vi "VCF.vi"(7 "Amount":fxp<+,8,0>, 9 "Q1":fxp<+/-,18,18>, 10 "F1":fxp<+/-,18,18>, 11 "Sample In":fxp<+/-,8,8>) -> (1 "BP Out":fxp<+/-,8,8>, 2 "LP Out":fxp<+/-,8,8>, 3 "HP Out":fxp<+/-,8,8>)   [LabVIEW 2015]
doc: "Executes simultaneous LP, HP and BP point-by-point filtering, being able to modify both the cutoff frequency and the resonance at run time. It also enables growl control, by routing an envelope generator output to the 'Amount' input."
uses:
  <vilib>/rvi/FXPMathLib/basic elements/DSP48E/simVIs/niFpgaDsp48eSimulationState.ctl
  <vilib>/rvi/FXPMathLib/basic elements/DSP48E/subVIs/niFpgaDsp48eType.ctl
  <vilib>/rvi/FXPMathLib/basic elements/DSP48E/subVIs/niFpgaDsp48eAlumodeOpmodeCarryinselState.ctl
  <vilib>/rvi/FXPMathLib/basic elements/DSP48E/subVIs/niFpgaDsp48eUseMultiplierState.ctl
  <vilib>/rvi/FXPMathLib/basic elements/DSP48E/subVIs/niFpgaDsp48eLogicUnitModeState.ctl
  <vilib>/rvi/FXPMathLib/basic elements/DSP48E/subVIs/niFpgaDsp48eSelectPatternState.ctl
  <vilib>/rvi/FXPMathLib/basic elements/DSP48E/subVIs/niFpgaDsp48eSelectMaskState.ctl
  <vilib>/rvi/FXPMathLib/basic elements/DSP48E/subVIs/niFpgaDsp48eAutoresetState.ctl
  <vilib>/rvi/FXPMathLib/basic elements/DSP48E/simVIs/niFpgaDsp48eResets.ctl
  <vilib>/rvi/FXPMathLib/basic elements/DSP48E/simVIs/niFpgaDsp48eEnables.ctl
  <vilib>/rvi/FXPMathLib/basic elements/DSP48E/simVIs/niFpgaDsp48eRegisters.ctl
  <vilib>/rvi/FXPMathLib/basic elements/DSP48E/simVIs/niFpgaDsp48eCheckMode.vi
  <vilib>/rvi/FXPMathLib/basic elements/DSP48E/simVIs/niFpgaDsp48eReportInvalidMode.vi
  <vilib>/rvi/FXPMathLib/basic elements/DSP48E/simVIs/niFpgaDsp48eSimMultiplier.vi
  <vilib>/rvi/FXPMathLib/basic elements/DSP48E/simVIs/niFpgaDsp48eSimArithmetic.vi
  <vilib>/rvi/FXPMathLib/basic elements/DSP48E/simVIs/niFpgaDsp48eSimPatternDetect.vi
  <vilib>/rvi/FXPMathLib/basic elements/DSP48E/simVIs/niFpgaDsp48eSimP.vi
  <vilib>/rvi/FXPMathLib/basic elements/DSP48E/simVIs/niFpgaDsp48eSimUpdateState.vi
  <vilib>/rvi/FXPMathLib/FxpMul/XNode/nifxpmath_Multiplier.xnode
  <vilib>/rvi/FXPMathLib/basic elements/DSP48E/XNode/niFpgaDsp48e.xnode
  <vilib>/rvi/FXPMathLib/sim/FxpSim.dll
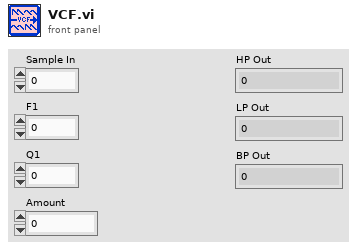
[diagram p1: front panel]
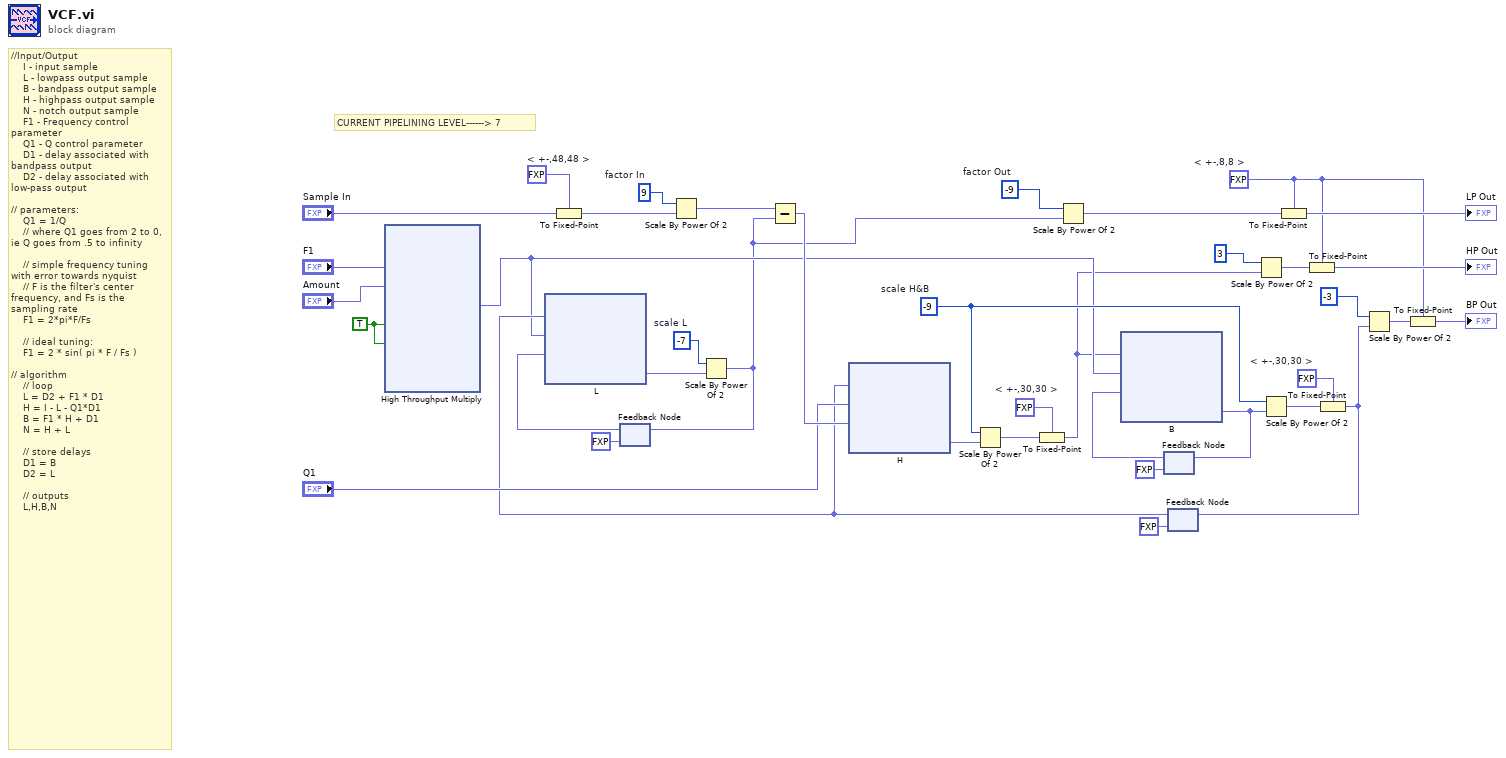
[diagram p0: block diagram]
diagram:
  w16 = TRUE ("input valid")
  w11 = i16 -9  # factor Out
  w19 = i16 -9  # scale H&B
  w32 = i16 -7  # scale L
  w30 = i16 9  # factor In
  w22 = fxp<+/-,30,30> 0.0  # < +-,30,30 >
  w24 = fxp<+/-,30,30> 0.0  # < +-,30,30 >
  w38 = fxp<+/-,48,48> 0.0  # < +-,48,48 >
  w1 = fxp<+/-,8,8> 0.0  # < +-,8,8 >
  # "CURRENT PIPELINING LEVEL------> 7"
  # "//Input/Output\n    I - input sample\n    L - lowpass output sample\n    B - bandpass output sample\n    H - highpass output sample\n    N - notch output sample\n    F1 - Frequency control parameter\n    Q1 - Q control parameter\n    D1 - delay associated with bandpass output\n    D2 - delay associated with low-pass output\n    \n// parameters:\n    Q1 = 1/Q \n    // where Q1 goes from 2 to 0, ie Q goes from .5 to infinity\n    \n    // simple frequency tuning with error towards nyquist\n    // F is the filter's center frequency, and Fs is the sampling rate\n    F1 = 2*pi*F/Fs\n\n    // ideal tuning:\n    F1 = 2 * sin( pi * F / Fs )\n\n// algorithm\n    // loop\n    L = D2 + F1 * D1\n    H = I - L - Q1*D1\n    B = F1 * H + D1\n    N = H + L\n    \n    // store delays\n    D1 = B\n    D2 = L\n\n    // outputs\n    L,H,B,N"
  n1 = xnode "High Throughput Multiply"("x"="F1", "y"="Amount", "input valid"=w16, "ready for output (T)"=w16) -> ("x*y"=w17:fxp<+/-,18,18>)  [unwired: 2 out]
  n2 = To Fixed-Point(fixed-point type=w38, number="Sample In") -> (fixed-point=w36:fxp<+/-,48,48>)
  n3 = feedback #1(fxp<+/-,48,48> 1.0) -> (w34:fxp<+/-,48,48>)
  n4 = Scale By Power Of 2(n=w30, x=w36) -> (x*2^n=w31:fxp<+/-,48,48>)
  n5 = feedback #2(fxp<+/-,48,48> 1.0 ("p")) -> (w27:fxp<+/-,48,48>)
  n6 = feedback #3(fxp<+/-,30,30> 1.0 ("< +-,30,30 >")) -> (w23:fxp<+/-,30,30>)
  n7 = xnode "L"("a"=w23, "b"=w17, "c"=w34) -> ("p"=w33:fxp<+/-,48,48>)
  n8 = Scale By Power Of 2(n=w32, x=w33) -> (x*2^n=w12:fxp<+/-,48,48>)
  n9 = feedback-in #1(w12) -> ()
  n10 = Subtract(x=w31, y=w12) -> (x-y=w29:fxp<+/-,48,48>)
  n11 = xnode "H"("a"=w23, "b"="Q1", "c"=w29) -> ("p"=w26:fxp<+/-,48,48>)
  n12 = Scale By Power Of 2(n=w19, x=w26) -> (x*2^n=w21:fxp<+/-,48,48>)
  n13 = To Fixed-Point(fixed-point type=w22, number=w21) -> (fixed-point=w7:fxp<+/-,30,30>)
  n14 = Scale By Power Of 2(n=w11, x=w12) -> (x*2^n=w18:fxp<+/-,48,48>)
  n15 = xnode "B"("a"=w7, "b"=w17, "c"=w27) -> ("p"=w20:fxp<+/-,48,48>)
  n16 = feedback-in #2(w20) -> ()
  n17 = Scale By Power Of 2(n=i16 3, x=w7) -> (x*2^n=w8:fxp<+/-,30,30>)
  n18 = Scale By Power Of 2(n=w19, x=w20) -> (x*2^n=w25:fxp<+/-,48,48>)
  n19 = To Fixed-Point(fixed-point type=w1, number=w18) -> (fixed-point=→"LP Out":fxp<+/-,8,8>)
  n20 = To Fixed-Point(fixed-point type=w1, number=w8) -> (fixed-point=→"HP Out":fxp<+/-,8,8>)
  n21 = To Fixed-Point(fixed-point type=w24, number=w25) -> (fixed-point=w5:fxp<+/-,30,30>)
  n22 = feedback-in #3(w5) -> ()
  n23 = Scale By Power Of 2(n=i16 -3, x=w5) -> (x*2^n=w3:fxp<+/-,30,30>)
  n24 = To Fixed-Point(fixed-point type=w1, number=w3) -> (fixed-point=→"BP Out":fxp<+/-,8,8>)
